vi "BLED1112-Set interval to min.vi"(2 "에러 입력(에러 없음)":errorcluster, 3 "VISA 리소스 이름":refnum<visa-resource-name>) -> (0 "에러 출력":errorcluster, 1 "VISA 리소스 이름 출력":refnum<visa-resource-name>)   [LabVIEW 2015]
panel:
  # "Set intervaltime to min."
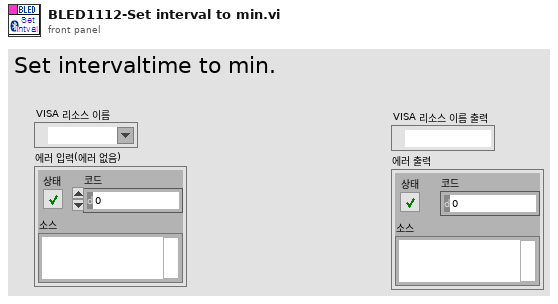
[diagram p1: front panel]
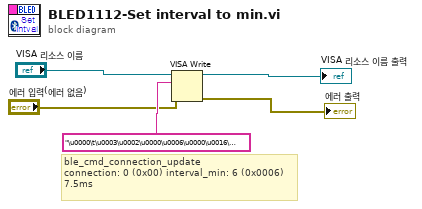
[diagram p0: block diagram]
diagram:
  # "ble_cmd_connection_update \nconnection: 0 (0x00) interval_min: 6 (0x0006)\n7.5ms"
  n1 = VISA Write(VISA resource name="VISA 리소스 이름", write buffer="\u0000\t\u0003\u0002\u0000\u0006\u0000\u0016\u0000\u0000\u0000d\u0000", error in (no error)="에러 입력(에러 없음)") -> (VISA resource name out=→"VISA 리소스 이름 출력":refnum<visa-resource-name>, error out=→"에러 출력":errorcluster)  [unwired: 1 out]
